vi "DHE_GetInitCmdLine.vi"(8 "link":string, 9 "devno":i32, 10 "type":string, 11 "fpa in":string) -> (0 "link out":string, 1 "devno out":i32, 2 "type out":string, 3 "fpa out":string)   [LabVIEW 2016]
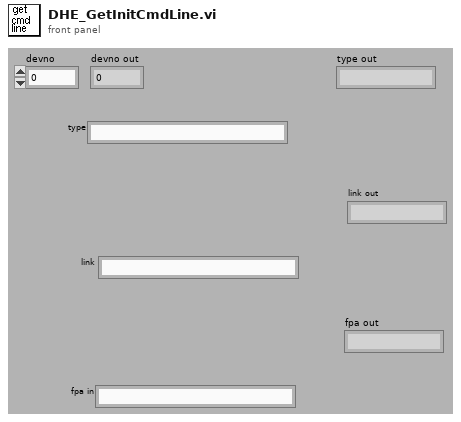
[diagram p1: front panel]
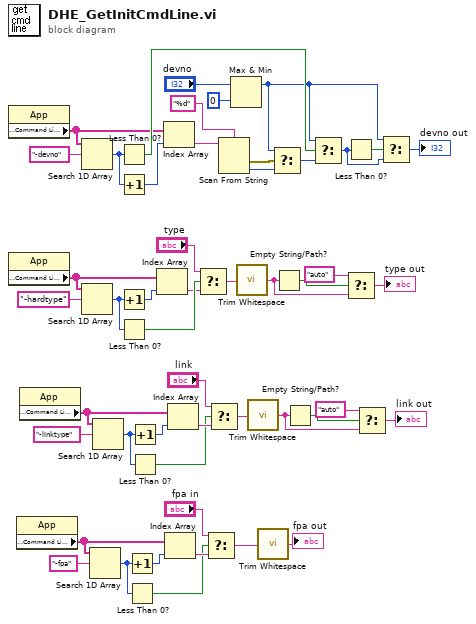
[diagram p0: block diagram]
diagram:
  n1 = property class="App"() -> ("Application:Command Line Arguments"=w35:string[])  [unwired: 2 in, 2 out]
  n2 = property class="App"() -> ("Application:Command Line Arguments"=w46:string[])  [unwired: 2 in, 2 out]
  n3 = property class="App"() -> ("Application:Command Line Arguments"=w8:string[])  [unwired: 2 in, 2 out]
  n4 = property class="App"() -> ("Application:Command Line Arguments"=w13:string[])  [unwired: 2 in, 2 out]
  n5 = Search 1D Array(1D array=w35, element="-devno") -> (index of element=w34:i32)  [unwired: 1 out]
  n6 = Search 1D Array(1D array=w46, element="-hardtype") -> (index of element=w45:i32)  [unwired: 1 out]
  n7 = Search 1D Array(1D array=w8, element="-fpa") -> (index of element=w7:i32)  [unwired: 1 out]
  n8 = Search 1D Array(1D array=w13, element="-linktype") -> (index of element=w14:i32)  [unwired: 1 out]
  n9 = Less Than 0?(x=w34) -> (x < 0?=w36:bool)
  n10 = Increment(x=w34) -> (x+1=w33:i32)
  n11 = Increment(x=w45) -> (x+1=w43:i32)
  n12 = Less Than 0?(x=w45) -> (x < 0?=w48:bool)
  n13 = Increment(x=w7) -> (x+1=w5:i32)
  n14 = Less Than 0?(x=w7) -> (x < 0?=w4:bool)
  n15 = Increment(x=w14) -> (x+1=w16:i32)
  n16 = Less Than 0?(x=w14) -> (x < 0?=w11:bool)
  n17 = Index Array(array=w46, index=w43) -> (element=w44:string)
  n18 = Index Array(array=w35, index=w33) -> (element=w32:string)
  n19 = Index Array(array=w8, index=w5) -> (element=w6:string)
  n20 = Index Array(array=w13, index=w16) -> (element=w15:string)
  n21 = Select(t="type", s=w48, f=w44) -> (s? t:f=w47:string)
  n22 = Select(t="fpa in", s=w4, f=w6) -> (s? t:f=w2:string)
  n23 = Select(t="link", s=w11, f=w15) -> (s? t:f=w12:string)
  n24 = Scan From String(format string="%d", input string=w32) -> (error out=w30:errorcluster, output 1=w29:i32)  [unwired: 2 in, 3 out]
  n25 = Max & Min(x="devno", y=0) -> (max(x,y)=w22:i32)  [unwired: 1 out]
  n26 = call <vilib>:"Trim Whitespace.vi"("string"=w47) -> ("trimmed string"=w41:string)  [unwired: 1 in]
  n27 = call <vilib>:"Trim Whitespace.vi"("string"=w12) -> ("trimmed string"=w18:string)  [unwired: 1 in]
  n28 = call <vilib>:"Trim Whitespace.vi"("string"=w2) -> ("trimmed string"=→"fpa out":string)  [unwired: 1 in]
  n29 = Select(t=w22, s=w30, f=w29) -> (s? t:f=w28:i32)
  n30 = Empty String/Path?(string/path=w41) -> (empty?=w42:bool)
  n31 = Empty String/Path?(string/path=w18) -> (empty?=w17:bool)
  n32 = Select(t=w22, s=w36, f=w28) -> (s? t:f=w26:i32)
  n33 = Less Than 0?(x=w26) -> (x < 0?=w27:bool)
  n34 = Select(t="auto", s=w42, f=w41) -> (s? t:f=→"type out":string)
  n35 = Select(t="auto", s=w17, f=w18) -> (s? t:f=→"link out":string)
  n36 = Select(t=w22, s=w27, f=w26) -> (s? t:f=→"devno out":i32)
